vi "Configure Frequency Voltage Range [FVR] Core.vi"(8 "error in (no error)":errorcluster, 10 "freq volt range (10.0 V RMS)":dbl=10.0 format="%^.2e", 11 "CS++DMM in":refnum<class "CS++DMM.lvclass">) -> (0 "error out":errorcluster, 3 "CS++DMM out":refnum<class "CS++DMM.lvclass">)   [LabVIEW 2015, in "CS++DMM.lvlib" / "CS++DMM.lvclass"]
doc: "This VI configures the frequency voltage range of the DMM for frequency and period measurements.\n\nThis VI affects the behavior of the instrument only if the IviDmm>Basic Operation>Function property is set to IVIDMM_VAL_FREQ or IVIDMM_VAL_PERIOD. \n\nNote:\n\n(1) This VI is part of the IviDmmFrequencyMeasurement [FRQ] extension group."
uses:
  CS++DMM.lvclass
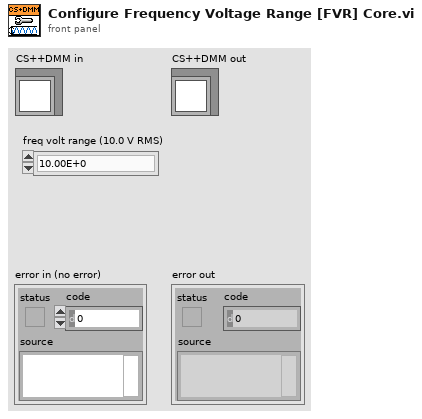
[diagram p1: front panel]
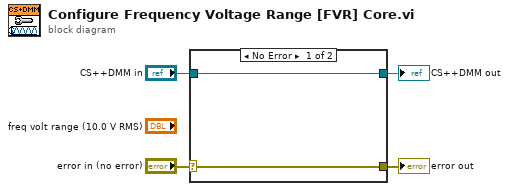
[diagram p0: block diagram]
diagram:
  n1 = case shown="No Error" "error in (no error)" {
    selector: "error in (no error)" -> [w5 w8]
    tunnel: [w5 w8] -> w3
    tunnel: [w6 w7] -> w1
    tunnel: "CS++DMM in" -> [w6 w7]
    frame No Error {
    }
    frame Error {
    }
  }
  "error out" <- w3
  "CS++DMM out" <- w1
